vi "to_json.vi"(8 "error in":errorcluster, 11 "gcs in":refnum<class "gcs.lvclass">) -> (0 "error out":errorcluster, 2 "json":string, 3 "gcs out":refnum<class "gcs.lvclass">)   [LabVIEW 2020, in "datasources.lvlib" / "gcs.lvclass"]
uses:
  gcs.lvclass
  C:/code/labview-client/lv_src/Nominal Client/datasources/source/source.lvclass
  source/source.lvclass/source.ctl
  e4c6944f-4a67-449d-9f92-17c70d7df472.vi
  source/path.get.vi
  <vilib>/JDP Science/JSONtext/Variant to JSON Text.vi
  <vilib>/JDP Science/JSONtext/LVClass Serializer/JSONtext LVClass Serializer.lvclass
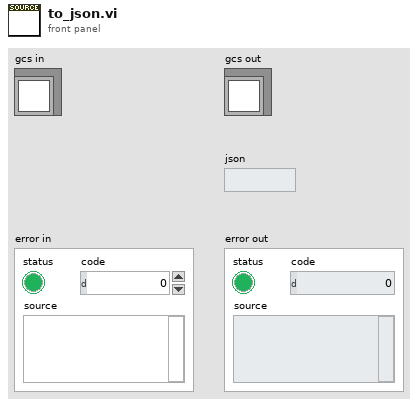
[diagram p1: front panel]
types:
  T1 = cluster{"type":string, "gcs":cluster{"path":string}}
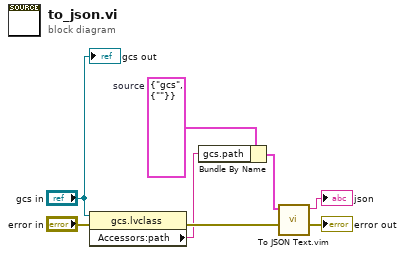
[diagram p0: block diagram]
diagram:
  w8 = T1 {"type"="gcs", "gcs"={"path"=""}}  # source
  n1 = property class="gcs.lvclass"(reference="gcs in", error in="error in") -> (error out=w6:errorcluster, "Accessors:path"=w5:string)  [unwired: 1 out]
  n2 = Bundle By Name(cluster=w8, "gcs.path"=w5) -> (w7:T1)
  n3 = call "To JSON Text.vim"("error in (no error)"=w6, "Anything"=w7) -> ("error out"=→"error out":errorcluster, "<JSON>"=→"json":string)  [unwired: 8 in]
  "gcs out" <- "gcs in"
